vi "Switch.vi"(6 "Channel List(empty)":string, 7 "Set/Check (F:Set)":bool, 8 "error in (no error)":errorcluster, 9 "Close Exclusive (F:Normal)":bool, 10 "Open/Close (F:Close)":bool, 11 "VISA Resource Name":refnum<visa-resource-name>) -> (0 "error out":errorcluster, 2 "Channel State?":string, 3 "VISA Resource Name Out":refnum<visa-resource-name>)   [LabVIEW 2016, in "Agilent 34970.lvlib"]
doc: "This VI lets you open/close a list of channels, such as those on the HP switching modules."
uses:
  Agilent 34970.lvlib
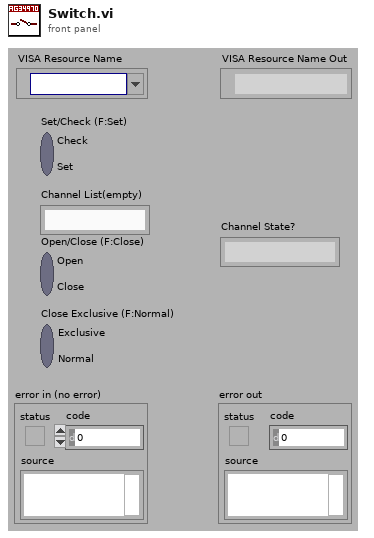
[diagram p1: front panel]
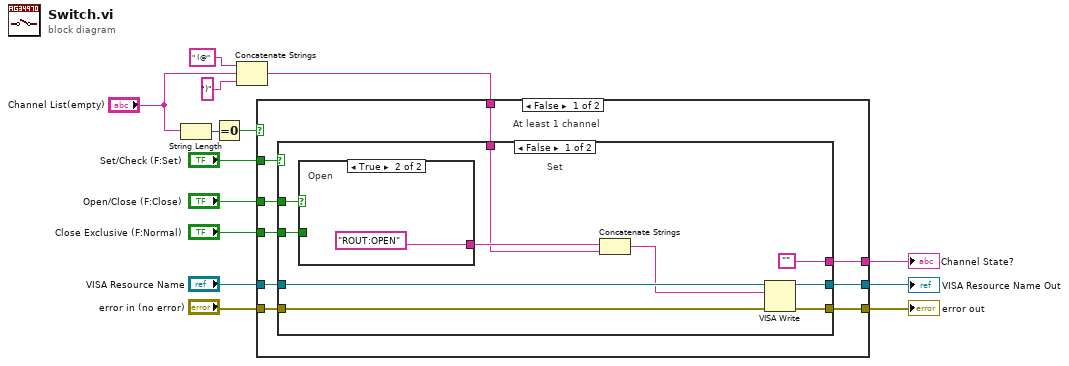
[diagram p0: block diagram]
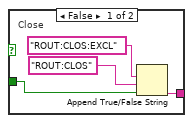
[diagram p2: hidden frame]
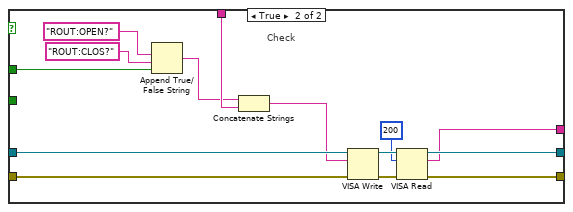
[diagram p3: hidden frame]
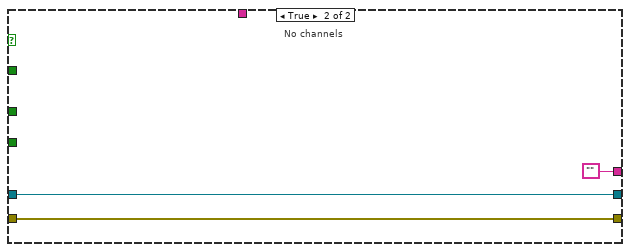
[diagram p4: hidden frame]
diagram:
  n1 = String Length(string="Channel List(empty)") -> (length=w7:i32)
  n2 = Equal To 0?(x=w7) -> (x = 0?=w9:bool)
  n3 = Concatenate Strings(" (@", "Channel List(empty)", ")") -> (w8:string)
  n4 = case shown="False" w9 {
    tunnel: [w23 ""] -> w10
    tunnel: [w22 w54] -> w2
    tunnel: [w21 w55] -> w1
    tunnel: "error in (no error)" -> [w20 w54]
    tunnel: "VISA Resource Name" -> [w19 w55]
    tunnel: w8 -> [w18 _]
    tunnel: "Close Exclusive (F:Normal)" -> [w17 _]
    tunnel: "Open/Close (F:Close)" -> [w16 _]
    tunnel: "Set/Check (F:Set)" -> [w15 _]
    frame False {
      # "At least 1 channel"
      n5 = case shown="False" w15 {
        tunnel: w16 -> [w33 w51]
        tunnel: w17 -> [w32 _]
        tunnel: w18 -> [w30 w49]
        tunnel: w19 -> [w29 w42]
        tunnel: w20 -> [w28 w41]
        tunnel: [w27 w47] -> w21
        tunnel: [w26 w45] -> w22
        tunnel: ["" w46] -> w23
        frame False {
          # "Set"
          n6 = case shown="True" w33 {
            tunnel: w32 -> [w37 _]
            tunnel: [w34 "ROUT:OPEN"] -> w31
            frame False {
              # "Close"
              n7 = Append True/False String(1:w37, 2:"ROUT:CLOS", 3:"ROUT:CLOS:EXCL") -> (0:w34:string)  [unwired: 1 in]
            }
            frame True {
              # "Open"
            }
          }
          n8 = Concatenate Strings(w31, w30) -> (w24:string)
          n9 = VISA Write(VISA resource name=w29, write buffer=w24, error in (no error)=w28) -> (VISA resource name out=w27:refnum<visa-resource-name>, error out=w26:errorcluster)  [unwired: 1 out]
        }
        frame True {
          # "Check"
          n10 = Append True/False String(1:w51, 2:"ROUT:CLOS?", 3:"ROUT:OPEN?") -> (0:w48:string)  [unwired: 1 in]
          n11 = Concatenate Strings(w48, w49) -> (w40:string)
          n12 = VISA Write(VISA resource name=w42, write buffer=w40, error in (no error)=w41) -> (VISA resource name out=w44:refnum<visa-resource-name>, error out=w43:errorcluster)  [unwired: 1 out]
          n13 = VISA Read(VISA resource name=w44, byte count=u32 200 ("byte count (0)"), error in (no error)=w43) -> (VISA resource name out=w47:refnum<visa-resource-name>, read buffer=w46:string, error out=w45:errorcluster)  [unwired: 1 out]
        }
      }
    }
    frame True {
      # "No channels"
    }
  }
  "Channel State?" <- w10
  "VISA Resource Name Out" <- w1
  "error out" <- w2
